vi "TalonFXCalibrateEncoder.vi"(0 "Device Reference (in)":T1={"DeviceStatus"={"status"=FALSE, "code"=0, "source"=""}, "Type"=enum."PWM", "PWM"={"PWM Channel"=enum."Invalid", "DeadBand"={"Name"="", "maxPositivePwm"=0, "minPositivePwm"=0, "centerPwm"=0, "maxNegativePwm"=0, "minNegativePwm"=0, "angularRange"=0}}, "CAN"={"Device Number"=0, "SetOutput VI Ref"=variant(enum8{"Percent VBus", "Current", "Speed", "Position", "Voltage"} enum."Percent VBus"), "GetOutput VI Ref"=variant(refnum<k1> refnum), "Enable VI Ref"=variant(dbl 12.0), "Disable VI Ref"=variant(enum8{"Percent VBus", "Speed", "Position", "Slave", "Unchanged / Invalid", "Voltage Compensation", "Current", "Motion Profile"} enum."Percent VBus"), "Data"=variant}, "Invert"=FALSE, "DIO PWM"={"PWM \"Enable\" Channel"=enum."Invalid", "DIOChannel"=enum."Invalid", "PWM Rate"=0.0}}, 1 "Gear Ratio":dbl=1.0, 5 "Calibration Trigger":bool, 9 "Calibration Angle (deg)":dbl, 11 "Error (in)":errorcluster) -> (4 "Device Reference (out)":T1, 10 "Currently Calibrating":bool, 15 "Error (out)":errorcluster)   [LabVIEW 2020]
doc: "Wrapper for calibrating the integrated relative encoders, using a specified calibration angle, on a Talon FX motor controller."
uses:
  <vilib>/Rock Robotics/WPI/MotorControl/WPI_MotorControlDeviceRef.ctl
  <vilib>/Rock Robotics/WPI/MotorControl/WPI_MotorControlType.ctl
  <vilib>/Rock Robotics/SystemInterfaces/DIO/FPGA_DIOPWMChannel.ctl
  <vilib>/Rock Robotics/WPI/PWM/WPI_PWMDeadband.ctl
  <vilib>/Rock Robotics/SystemInterfaces/DIO/FPGA_DIOChannel.ctl
  <vilib>/Rock Robotics/WPI/ThirdParty/Phoenix-LabVIEW/Motor Controller/Get/CTRE_Phoenix_MotorController_GetSelectedSensorData.vi
  <vilib>/Rock Robotics/WPI/ThirdParty/Phoenix-LabVIEW/Motor Controller/Get/CTRE_Phoenix_MotorController_GetGeneralStatus.vi
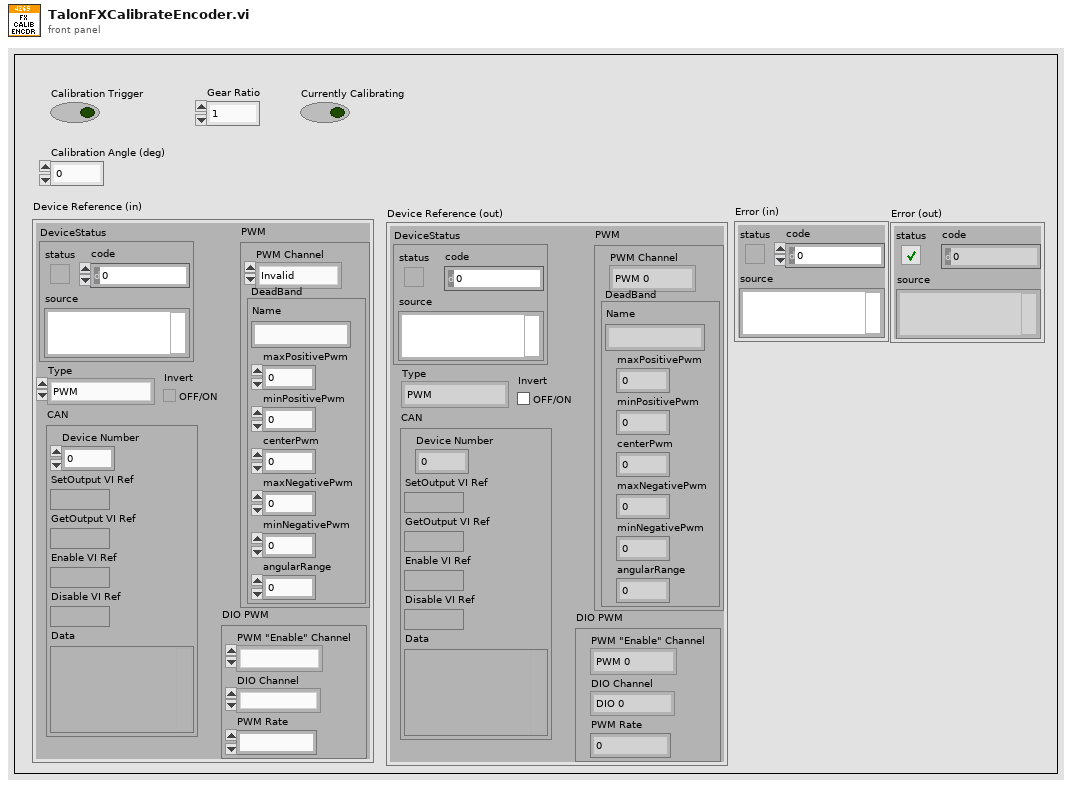
[diagram p1: front panel]
types:
  T1 = typedef "WPI_MotorControlDeviceRef.ctl" = cluster{"DeviceStatus":errorcluster, "Type":T2, "PWM":cluster{"PWM Channel":T3, "DeadBand":T4}, "CAN":cluster{"Device Number":u8, "SetOutput VI Ref":variant, "GetOutput VI Ref":variant, "Enable VI Ref":variant, "Disable VI Ref":variant, "Data":variant}, "Invert":bool, "DIO PWM":cluster{"PWM \"Enable\" Channel":T3, "DIOChannel":T5, "PWM Rate":dbl}}
  T2 = typedef "WPI_MotorControlType.ctl" = enum16{"PWM", "CAN", "DIO PWM"}
  T3 = typedef "FPGA_DIOPWMChannel.ctl" = enum8{"PWM 0", "PWM 1", "PWM 2", "PWM 3", "PWM 4", "PWM 5", "PWM 6", "PWM 7", "PWM 8", "PWM 9", "PWM MXP 0", "PWM MXP 1", "PWM MXP 2", "PWM MXP 3", "PWM MXP 4", "PWM MXP 5", "PWM MXP 6", "PWM MXP 7", "PWM MXP 8", "PWM MXP 9", "Invalid"}
  T4 = typedef "WPI_PWMDeadband.ctl" = cluster{"Name":string, "maxPositivePwm":i32, "minPositivePwm":i32, "centerPwm":i32, "maxNegativePwm":i32, "minNegativePwm":i32, "angularRange":u16}
  T5 = typedef "FPGA_DIOChannel.ctl" = enum8{"DIO 0", "DIO 1", "DIO 2", "DIO 3", "DIO 4", "DIO 5", "DIO 6", "DIO 7", "DIO 8", "DIO 9", "DIO MXP 0", "DIO MXP 1", "DIO MXP 2", "DIO MXP 3", "DIO MXP 4", "DIO MXP 5", "DIO MXP 6", "DIO MXP 7", "DIO MXP 8", "DIO MXP 9", "DIO MXP 10", "DIO MXP 11", "DIO MXP 12", "DIO MXP 13", "DIO MXP 14", "DIO MXP 15", "SPI Port CS1", "SPI Port CS2", "SPI Port CS3", "SPI Port MISO", "SPI Port MOSI", "Invalid"}
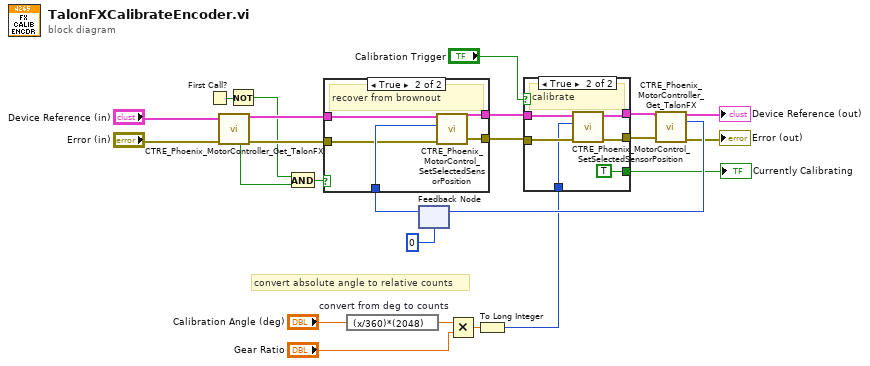
[diagram p0: block diagram]
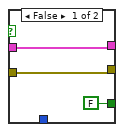
[diagram p2: hidden frame]
diagram:
  # "convert absolute angle to relative counts"
  n1 = First Call?() -> (First Call?: T/F=w13:bool)
  n2 = call-poly <vilib>:"CTRE_Phoenix_MotorController_Get_TalonFX.vi"("PhoenixMotorControlDevRef"="Device Reference (in)", "error in"="Error (in)") -> ("PhoenixMotorControlDevRef"=w15:T1, "Has Reset Occurred?"=w17:bool, "error out"=w16:errorcluster)  [unwired: 8 in, 3 out]
  n3 = Not(x=w13) -> (.not. x?=w14:bool)
  n4 = And(x=w14, y=w17) -> (x .and. y?=w12:bool)
  n5 = expression code="(x/360)*(2048)" "convert from deg to counts"("Calibration Angle (deg)") -> (w21:dbl)
  n6 = feedback #1(0 ("Position (Raw Sensor Units)")) -> (w9:i32)
  n7 = case shown="True" w12 {
    tunnel: w16 -> [w25 w29]
    tunnel: w15 -> [w26 w31]
    tunnel: [w26 w28] -> w10
    tunnel: [w25 w27] -> w11
    tunnel: w9 -> [_ w30]
    frame False {
    }
    frame True {
      # "recover from brownout"
      n8 = call <vilib>:"CTRE_Phoenix_MotorControl_SetSelectedSensorPosition.vi"("error in (no error)"=w29, "New Sensor Position"=w30, "PhoenixMotorControlDevRef"=w31) -> ("error out"=w27:errorcluster, "PhoenixMotorControlDevRef"=w28:T1)  [unwired: 7 in]
    }
  }
  n9 = Multiply(x=w21, y="Gear Ratio") -> (x*y=w22:dbl)
  n10 = To Long Integer(number=w22) -> (32bit integer=w5:i32)
  n11 = case shown="True" "Calibration Trigger" {
    tunnel: w11 -> [w33 w37]
    tunnel: w10 -> [w34 w38]
    tunnel: [w34 w39] -> w18
    tunnel: [w33 w40] -> w19
    tunnel: w5 -> [_ w36]
    tunnel: [FALSE TRUE] -> w1
    frame False {
    }
    frame True {
      # "calibrate"
      n12 = call <vilib>:"CTRE_Phoenix_MotorControl_SetSelectedSensorPosition.vi"("error in (no error)"=w37, "New Sensor Position"=w36, "PhoenixMotorControlDevRef"=w38) -> ("error out"=w40:errorcluster, "PhoenixMotorControlDevRef"=w39:T1)  [unwired: 7 in]
    }
  }
  "Currently Calibrating" <- w1
  n13 = call-poly <vilib>:"CTRE_Phoenix_MotorController_Get_TalonFX.vi"("PhoenixMotorControlDevRef"=w18, "error in"=w19) -> ("PhoenixMotorControlDevRef"=→"Device Reference (out)":T1, "Position (Raw Sensor Units)"=w20:i32, "error out"=→"Error (out)":errorcluster)  [unwired: 10 in, 1 out]
  n14 = feedback-in #1(w20) -> ()
